vi "is_empty.vi"(8 "error in (no error)":errorcluster, 11 "Image in":refnum<class "Image.lvclass">) -> (0 "error out":errorcluster, 2 "emtpy?":bool, 3 "Image out":refnum<class "Image.lvclass">)   [LabVIEW 2010, in "Image.lvclass"]
uses:
  Image.lvclass
  <vilib>/vision/Image Controls.llb/IMAQ Image.ctl
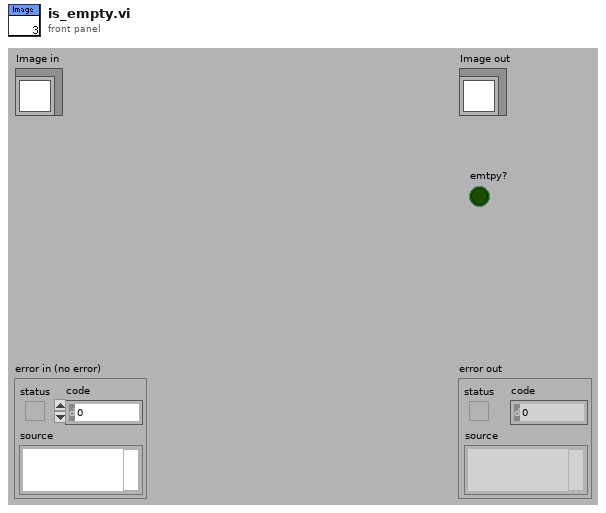
[diagram p1: front panel]
types:
  T1 = typedef "IMAQ Image.ctl" = refnum<image>
  T2 = typedef "Image.lvclass/storage_mode.ctl" = enum16{"RAM", "disk"}
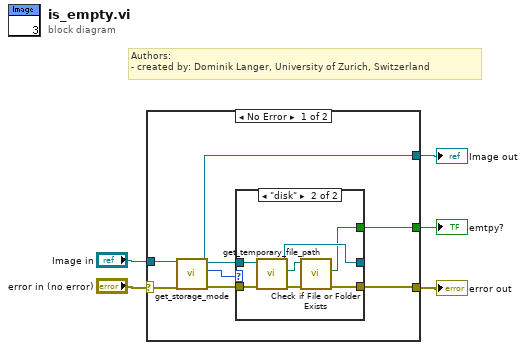
[diagram p0: block diagram]
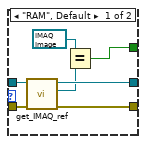
[diagram p2: hidden frame]
diagram:
  # "Authors: \n- created by: Dominik Langer, University of Zurich, Switzerland"
  n1 = case shown="No Error" "error in (no error)" {
    selector: "error in (no error)" -> [w12 w28]
    tunnel: [w7 w28] -> w4
    tunnel: [w8 w27] -> w2
    tunnel: "Image in" -> [w11 w27]
    tunnel: [w6 _] -> w1
    frame No Error {
      n2 = call-dynamic "get_storage_mode.vi"("error in (no error)"=w12, "Image.lvclass in"=w11) -> ("error out"=w9:errorcluster, "storage mode"=w10:T2, "Image.lvclass out"=w8:refnum<class "Image.lvclass">)  [unwired: 7 out]
      n3 = case shown="\"disk\"" w10 {
        tunnel: w9 -> [w19 w26]
        tunnel: w8 -> [w18 w25]
        tunnel: [w17 w24] -> _
        tunnel: [w16 w22] -> w7
        tunnel: [w13 w20] -> w6
        frame "RAM", Default {
          n4 = call-dynamic "get_IMAQ_ref.vi"("error in (no error)"=w19, "Image.lvclass in"=w18) -> ("error out"=w16:errorcluster, "Image"=w15:T1, "Image.lvclass out"=w17:refnum<class "Image.lvclass">)  [unwired: 7 out]
          n5 = Equal?(x=T1 refnum ("Image"), y=w15) -> (x = y?=w13:bool)
        }
        frame "disk" {
          n6 = call-dynamic "get_temporary_file_path.vi"("error in (no error)"=w26, "Image.lvclass in"=w25) -> ("error out"=w23:errorcluster, "temporary file path"=w21:path, "Image.lvclass out"=w24:refnum<class "Image.lvclass">)  [unwired: 7 out]
          n7 = call <vilib>:"Check if File or Folder Exists.vi"("error in (no error)"=w23, "path"=w21) -> ("error out"=w22:errorcluster, "file or folder exists?"=w20:bool)  [unwired: 8 out]
        }
      }
    }
    frame Error {
    }
  }
  "error out" <- w4
  "Image out" <- w2
  "emtpy?" <- w1
